vi "Array_Trans.vi"(0 "rohR [Ohm]":dbl[](array[numeric]), 1 "kappaR [A²]":dbl[](array[numeric]), 3 "Single Channel Voltage":dbl[](array[numeric]), 4 "rohM [Ohm]":dbl[](array[numeric]), 5 "tauR [s]":dbl[](array[numeric]), 7 "NSamples":i32, 8 "offset [V]":dbl[](array[numeric]), 9 "kappaM [A²]":dbl[](array[numeric]), 12 "full P_rad VBC":dbl[](array[numeric]), 13 "full P_rad HBC":dbl[](array[numeric]), 15 "tauM [s]":dbl[](array[numeric]), 18 "real time P_rad":dbl[](array[numeric])) -> (10 "full P_rad VBC":dbl[][](array[numeric]), 14 "Mean [mV]":dbl[][](array[numeric]), 16 "tauR [s]":dbl[][](array[numeric]), 17 "rohR [Ohm]":dbl[][](array[numeric]), 19 "real time P_rad":dbl[][](array[numeric]), 20 "tauM [s]":dbl[][](array[numeric]), 21 "kappa [A²]":dbl[][](array[numeric]), 23 "full P_rad HBC":dbl[][](array[numeric]), 24 "kappaR [A²]":dbl[][](array[numeric]), 25 "rohM [Ohm]":dbl[][](array[numeric]), 27 "Single Channel Voltage":dbl[][](array[numeric]))   [LabVIEW 2014]
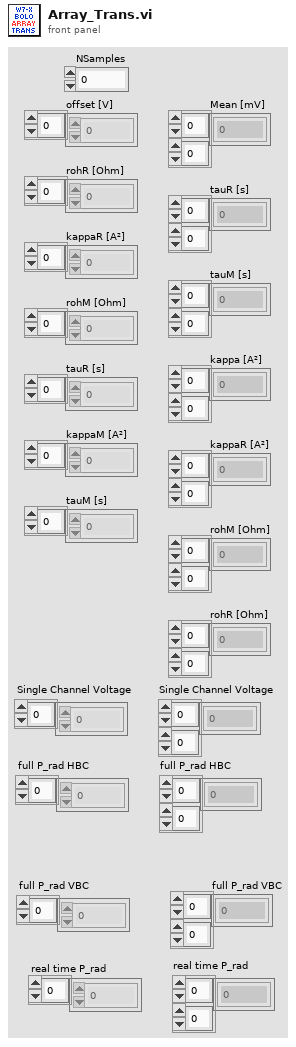
[diagram p1: front panel]
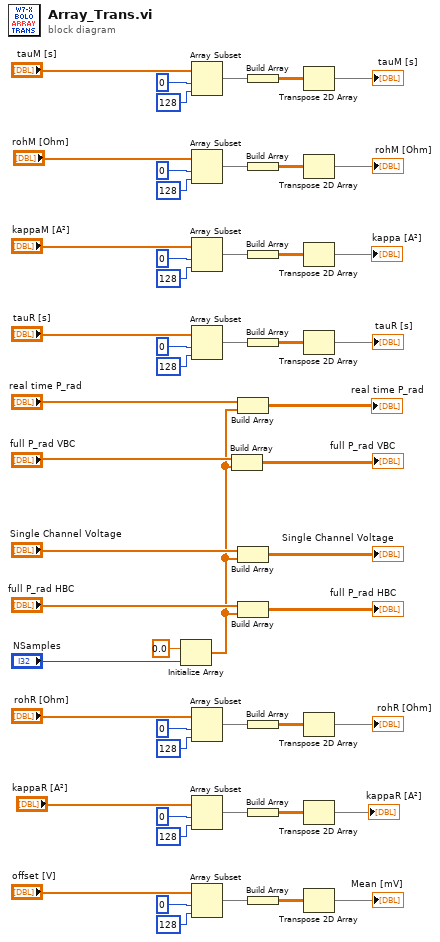
[diagram p0: block diagram]
diagram:
  n1 = Initialize Array(0.0 ("element"), "NSamples") -> (w3:dbl[])
  n2 = Array Subset(array="tauM [s]", index=0, length=128) -> (w50:dbl[])
  n3 = Array Subset(array="rohM [Ohm]", index=0, length=128) -> (w47:dbl[])
  n4 = Array Subset(array="kappaM [A²]", index=0, length=128) -> (w43:dbl[])
  n5 = Array Subset(array="tauR [s]", index=0, length=128) -> (w40:dbl[])
  n6 = Array Subset(array="rohR [Ohm]", index=0, length=128) -> (w38:dbl[])
  n7 = Array Subset(array="kappaR [A²]", index=0, length=128) -> (w35:dbl[])
  n8 = Array Subset(array="offset [V]", index=0, length=128) -> (w28:dbl[])
  n9 = Build Array("full P_rad VBC", w3) -> (→"full P_rad VBC":dbl[][])
  n10 = Build Array("real time P_rad", w3) -> (→"real time P_rad":dbl[][])
  n11 = Build Array("Single Channel Voltage", w3) -> (→"Single Channel Voltage":dbl[][])
  n12 = Build Array("full P_rad HBC", w3) -> (→"full P_rad HBC":dbl[][])
  n13 = Build Array(w50) -> (w49:dbl[][])
  n14 = Build Array(w47) -> (w46:dbl[][])
  n15 = Build Array(w43) -> (w44:dbl[][])
  n16 = Build Array(w40) -> (w41:dbl[][])
  n17 = Build Array(w38) -> (w37:dbl[][])
  n18 = Build Array(w35) -> (w36:dbl[][])
  n19 = Build Array(w28) -> (w32:dbl[][])
  n20 = Transpose 2D Array(2D array=w49) -> (transposed array=→"tauM [s]":dbl[][])
  n21 = Transpose 2D Array(2D array=w46) -> (transposed array=→"rohM [Ohm]":dbl[][])
  n22 = Transpose 2D Array(2D array=w44) -> (transposed array=→"kappa [A²]":dbl[][])
  n23 = Transpose 2D Array(2D array=w41) -> (transposed array=→"tauR [s]":dbl[][])
  n24 = Transpose 2D Array(2D array=w37) -> (transposed array=→"rohR [Ohm]":dbl[][])
  n25 = Transpose 2D Array(2D array=w36) -> (transposed array=→"kappaR [A²]":dbl[][])
  n26 = Transpose 2D Array(2D array=w32) -> (transposed array=→"Mean [mV]":dbl[][])
